vi "Advanced settings.vi"() -> (2 "output cluster":T2)   [LabVIEW 2011]
uses:
  Buttons/Numeric control.ctl
panel:
  in  "Log interval (HRS)":T1=300.0 min=0.0 max=3600.0 step=0.1
  in  "Purge duration (seconds)":T1=300.0 min=0.0 max=3600.0 step=1.0
  in  "lambda D":T1=0.0075 min=0.0 max=5.0 step=0.0001
  in  "lambda I":T1=10.0 min=0.0 max=10.0 step=0.01
  in  "lambda P":T1=3.0 min=0.0 max=10.0 step=0.01
  in  "OK Button 2":bool=TRUE
  in  "CRF HC %":T1=0.0075 min=0.0 max=5.0 step=0.0001
  in  "CO Factor 'O'":T1=10.0 min=0.0 max=10.0 step=0.01
  in  "CO Factor 'B'":T1=3.0 min=0.0 max=10.0 step=0.01
  in  "OK Button":bool
  in  "Bleed ratio CO2":T1=20.0 min=0.0 step=0.1
  in  "Bleed ratio N2":T1=19.0 min=0.0 step=0.1
  in  "NOx Concentration (ppm)":T1=35000.0 min=0.0 step=1.0
  in  "SO2 Concentration (ppm)":T1=20000.0 min=0.0 step=1.0
  in  "CO concentration %":T1=100.0 min=0.0 max=100.0 step=1.0
  in  "HC concentration %":T1=100.0 min=0.0 max=100.0 step=1.0
  # "Advanced settings"
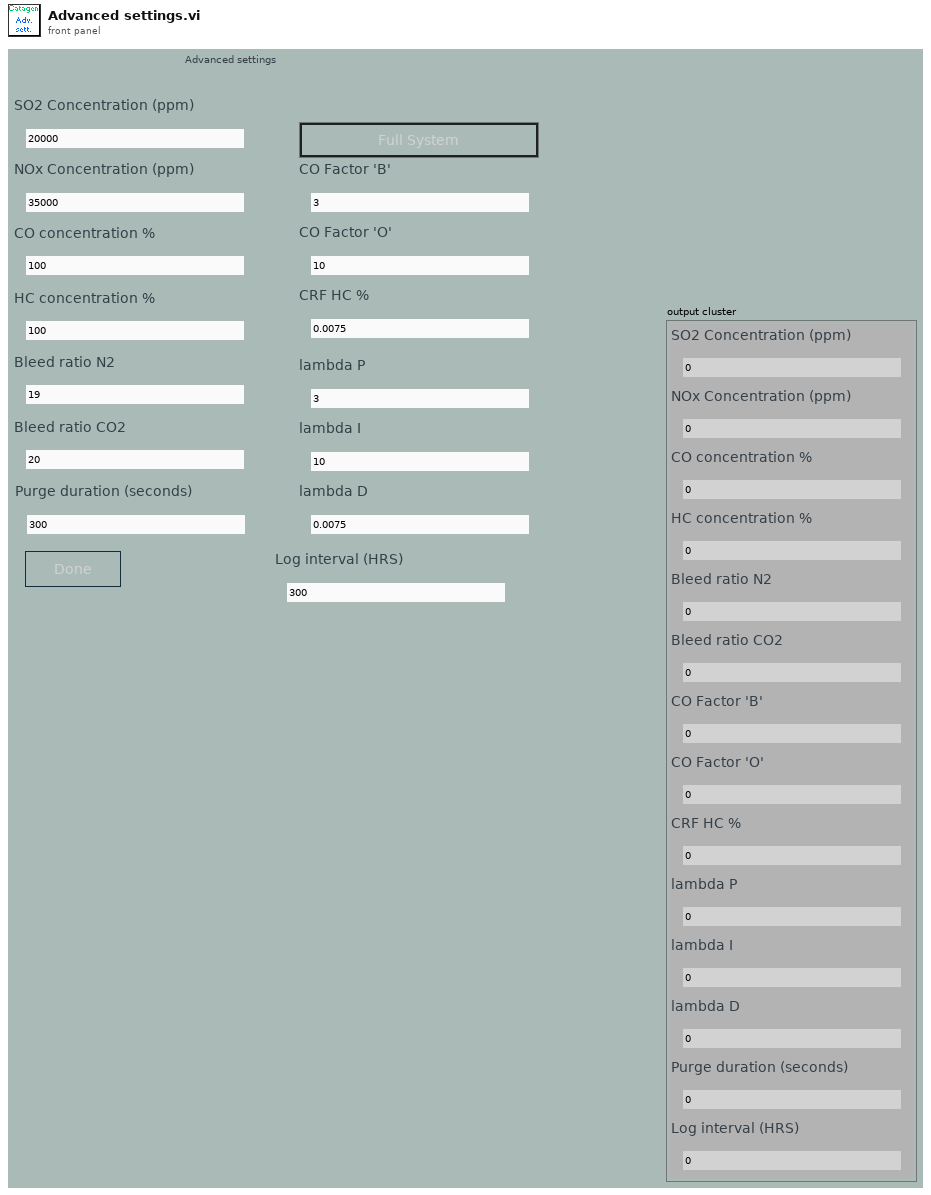
[diagram p1: front panel]
types:
  T1 = typedef "Numeric control.ctl" = dbl
  T2 = cluster{"SO2 Concentration (ppm)":T1, "NOx Concentration (ppm)":T1, "CO concentration %":T1, "HC concentration %":T1, "Bleed ratio N2":T1, "Bleed ratio CO2":T1, "CO Factor 'B'":T1, "CO Factor 'O'":T1, "CRF HC %":T1, "lambda P":T1, "lambda I":T1, "lambda D":T1, "Purge duration (seconds)":T1, "Log interval (HRS)":T1}
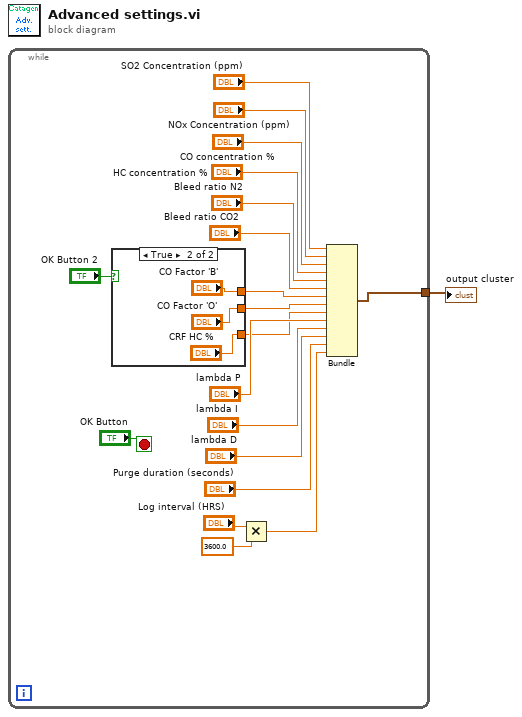
[diagram p0: block diagram]
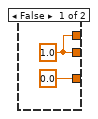
[diagram p2: hidden frame]
diagram:
  n1 = while {
    tunnel: [w13] -> w1
    stop <- "OK Button" stop-if-true
    n2 = case shown="True" "OK Button 2" {
      tunnel: [w22 "CO Factor 'B'"] -> w8
      tunnel: [w22 "CO Factor 'O'"] -> w7
      tunnel: [T1 0.0 ("CO Factor 'B'") "CRF HC %"] -> w6
      frame False {
        w22 = T1 1.0 ("CO Factor 'B'")
      }
      frame True {
      }
    }
    n3 = Multiply(x="Log interval (HRS)", y=T1 3600.0) -> (x*y=w2:T1)
    n4 = Bundle("SO2 Concentration (ppm)"="SO2 Concentration (ppm)", "NOx Concentration (ppm)"="NOx Concentration (ppm)", "CO concentration %"="CO concentration %", "HC concentration %"="HC concentration %", "Bleed ratio N2"="Bleed ratio N2", "Bleed ratio CO2"="Bleed ratio CO2", "CO Factor 'B'"=w8, "CO Factor 'O'"=w7, "CRF HC %"=w6, "lambda P"="lambda P", "lambda I"="lambda I", "lambda D"="lambda D", "Purge duration (seconds)"="Purge duration (seconds)", "Log interval (HRS)"=w2) -> (w13:T2)  [unwired: 1 in]
  }
  "output cluster" <- w1
